vi "CalNumOfDisplay.vi"(2 "IndexOfBase":u32, 3 "DataSum":u32) -> (1 "NumOfDisplay":u32)   [LabVIEW 2015, in "ActorManagement.lvlib" / "AdvanceTable.lvclass"]
uses:
  AdvanceTable.lvclass
  Config/g_tabSetting.vi
  ActorManagement.lvlib
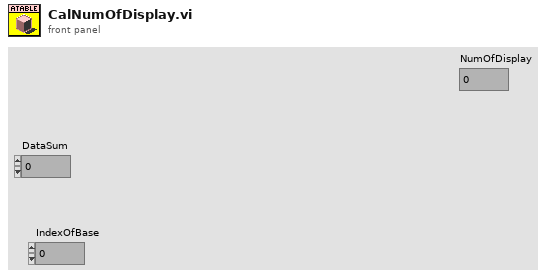
[diagram p1: front panel]
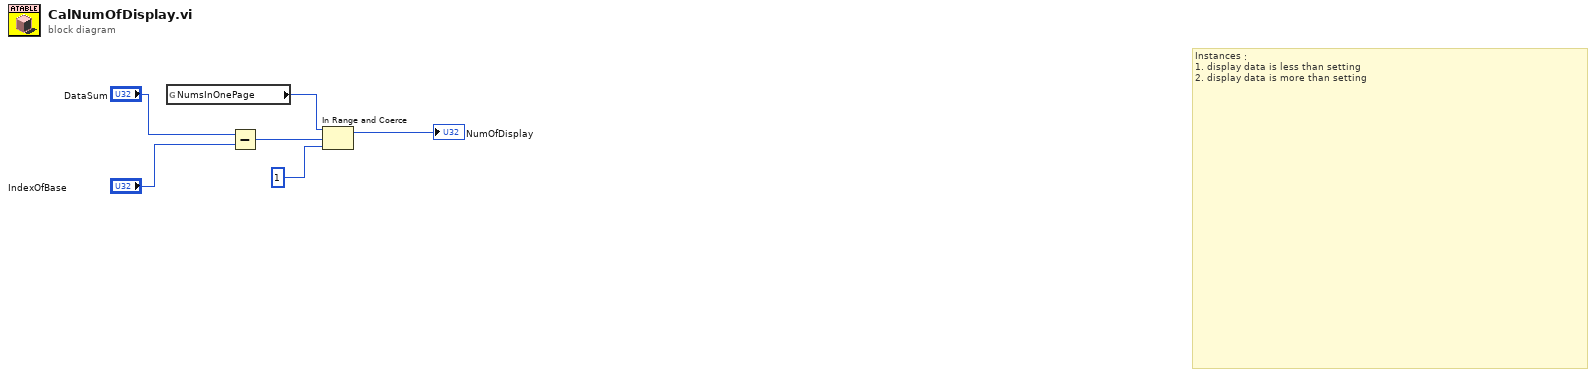
[diagram p0: block diagram]
diagram:
  # "Instances：\n1. display data is less than setting \n2. display data is more than setting"
  n1 = global read "g_tabSetting.vi" "NumsInOnePage"() -> (w3:u32)
  n2 = Subtract(x="DataSum", y="IndexOfBase") -> (x-y=w4:u32)
  n3 = In Range and Coerce(upper limit=w3, x=w4, lower limit=u32 1) -> (coerced(x)=→"NumOfDisplay":u32)  [unwired: 1 out]
